vi "Cleanup.vi"(8 "error in (no error)":errorcluster, 11 "Item Summary in":refnum<class "Item Summary.lvclass">) -> (0 "error out":errorcluster)   [LabVIEW 2020, in "Item Summary.lvclass"]
uses:
  Item Summary.lvclass
  <vilib>/IlluminatedG/IG OOPanel/OOPanel/ArrayPanel/ArrayPanel.lvclass
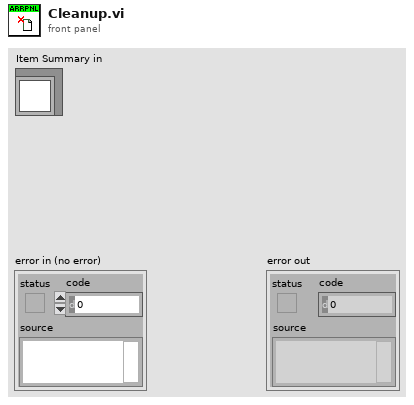
[diagram p1: front panel]
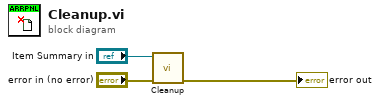
[diagram p0: block diagram]
diagram:
  n1 = call-parent "Cleanup.vi"("error in (no error)"="error in (no error)", "ArrayPanel in"="Item Summary in") -> ("error out"=→"error out":errorcluster)  [unwired: 9 in]
